vi "CreateNanosecondTimestamp.vi"(11 "current time":timestamp) -> (2 "Timestring in RFC3339Nano":string, 3 "Time in RFC3339Nano":i64)   [LabVIEW 2019, in "hse-logger.lvlib" / "LokiJsonFormatter.lvclass"]
doc: "Excerpt from official documentation on how they are interpreted:\n\nThe API accepts several formats for timestamps. An integer with ten or fewer digits is interpreted as a Unix timestamp in seconds. More than ten digits are interpreted as a Unix timestamp in nanoseconds. A floating point number is a Unix timestamp with fractions of a second.\n\nThe timestamps can also be written in RFC3339 and RFC3339Nano format, as supported by Go’s time package."
uses:
  LokiJsonFormatter.lvclass
panel:
  # "Connector Pane"
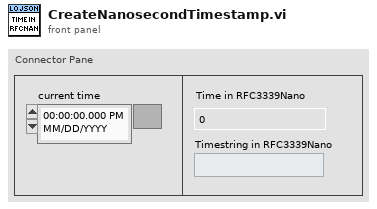
[diagram p1: front panel]
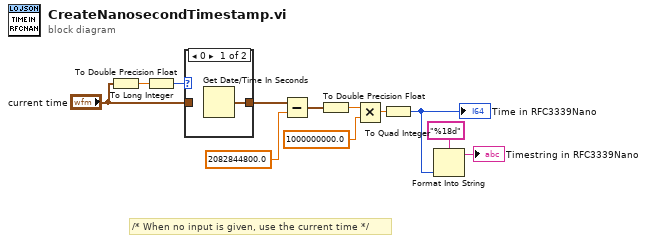
[diagram p0: block diagram]
diagram:
  # "/* When no input is given, use the current time */"
  n1 = To Double Precision Float(number="current time") -> (double precision float=w12:dbl)
  n2 = To Long Integer(number=w12) -> (32bit integer=w11:i32)
  n3 = case shown="0" w11 {
    tunnel: [w13 w14] -> w6
    tunnel: "current time" -> [_ w14]
    frame 0 {
      n4 = Get Date/Time In Seconds() -> (seconds since 1Jan1904=w13:timestamp)
    }
    frame Default {
    }
  }
  n5 = Subtract(x=w6, y=2082844800.0) -> (x-y=w9:timestamp)
  n6 = To Double Precision Float(number=w9) -> (double precision float=w10:dbl)
  n7 = Multiply(x=w10, y=1000000000.0) -> (x*y=w4:dbl)
  n8 = To Quad Integer(1:w4) -> (0:w1:i64)
  "Time in RFC3339Nano" <- w1
  n9 = Format Into String(format string="%18d", w1) -> (resulting string=→"Timestring in RFC3339Nano":string)  [unwired: 2 in, 1 out]
